vi "Check if Any File Exists.vi"(0 "File Directory":path, 5 "File Names":string[](array[string])=["Gameover.txt", "input_%d.txt"], 7 "Play Number":i32, 11 "error in (no error)":errorcluster) -> (4 "File Found?":bool, 6 "Found File":path, 8 "Game Over?":bool, 15 "error out":errorcluster)   [LabVIEW 2014, in "Dragon Tamers.lvlib"]
uses:
  Dragon Tamers.lvlib
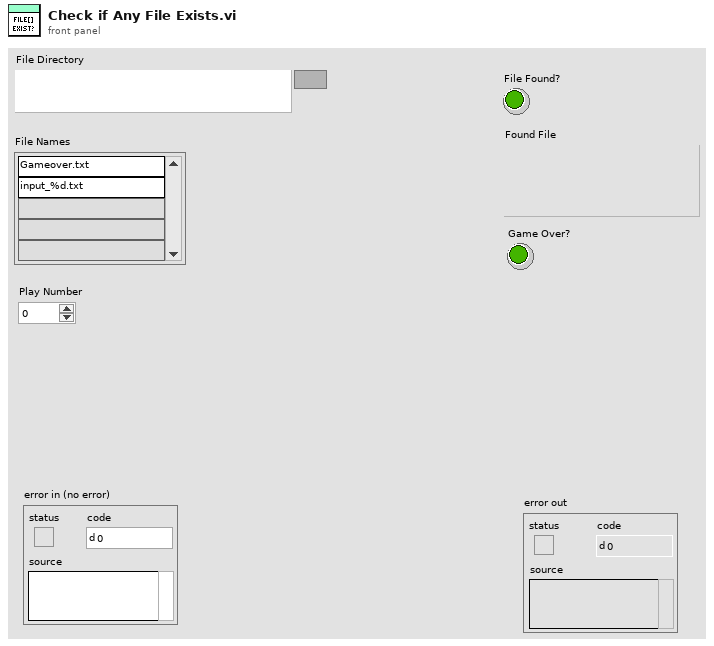
[diagram p1: front panel]
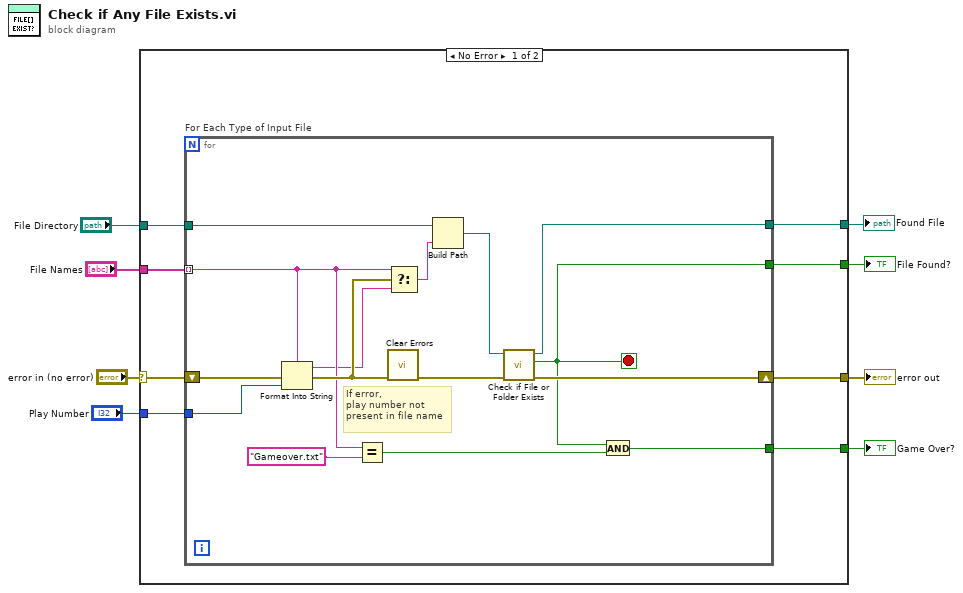
[diagram p0: block diagram]
diagram:
  n1 = case shown="No Error" "error in (no error)" {
    selector: "error in (no error)" -> [w16 w32]
    tunnel: "File Names" -> [w14 _]
    tunnel: "Play Number" -> [w15 _]
    tunnel: "File Directory" -> [w13 _]
    tunnel: [w12 _] -> w1
    tunnel: [w11 w32] -> w4
    tunnel: [w10 _] -> w3
    tunnel: [w9 _] -> w2
    frame No Error {
      n2 = for "For Each Type of Input File" {
        tunnel: w15 -> [w30]
        tunnel: w14 -> [w20] mode=indexing
        tunnel: w13 -> [w24]
        shift-right: [w29] -> w11
        shift-left: w16 -> [w31]
        tunnel: [w28] -> w12
        tunnel: [w26] -> w10
        tunnel: [w25] -> w9
        stop <- w26 stop-if-true
        # "If error,\nplay number not\npresent in file name"
        n3 = Format Into String(format string=w20, error in=w31, w30) -> (resulting string=w19:string, error out=w21:errorcluster)  [unwired: 1 in]
        n4 = Equal?(x=w20, y="Gameover.txt") -> (x = y?=w22:bool)
        n5 = call <vilib>:"Clear Errors.vi"("error in (no error)"=w21) -> ("error out"=w17:errorcluster)  [unwired: 5 in, 1 out]
        n6 = Select(t=w20, s=w21, f=w19) -> (s? t:f=w18:string)
        n7 = Build Path(base path=w24, name or relative path=w18) -> (appended path=w23:path)
        n8 = call <vilib>:"Check if File or Folder Exists.vi"("error in (no error)"=w17, "path"=w23) -> ("error out"=w29:errorcluster, "file or folder exists?"=w26:bool, "dup path"=w28:path)  [unwired: 7 in]
        n9 = And(x=w26, y=w22) -> (x .and. y?=w25:bool)
      }
    }
    frame Error {
    }
  }
  "error out" <- w4
  "File Found?" <- w3
  "Game Over?" <- w2
  "Found File" <- w1
